vi "TDMS Read Telemtry Data.vi"() -> ()   [LabVIEW 2021]
doc: "This example demonstrates how to read measured data, text and timestamps from a .tdms file using the TDMS API."
panel:
  out "Measured Data":waveform(dbl)[](graph)
  in  "Event Data":i32(listbox)=-1
  # "Overview: Demonstrates the use of the TDMS Read function to read measured data, text and timestamps from an existing .tdms file.\nInstructions:\n1. Make sure you have already run TDMS Write Events Data.vi.\n2. Run this VI.\n3. Delete the .tdms file (located at [LabVIEW Data]\\Example Events Data.tdms) when you are done."
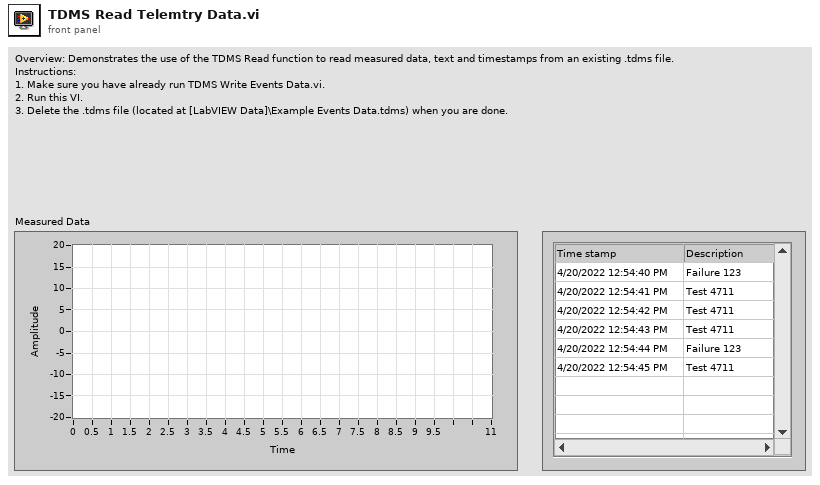
[diagram p1: front panel]
types:
  T1 = enum16{"open", "open or create", "create or replace", "create", "open (read-only)"}
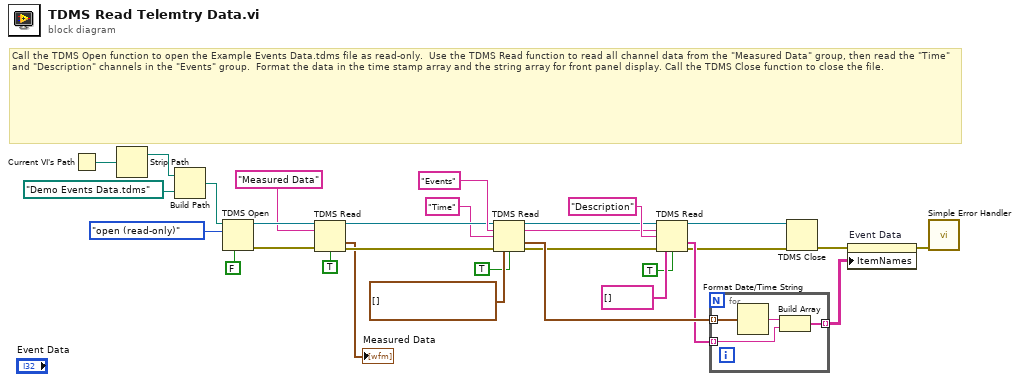
[diagram p0: block diagram]
diagram:
  # "Call the TDMS Open function to open the Example Events Data.tdms file as read-only.  Use the TDMS Read function to read all channel data from the \"Measured Data\" group, then read the \"Time\" and \"Description\" channels in the \"Events\" group.  Format the data in the time stamp array and the string array for front panel display. Call the TDMS Close function to close the file."
  n1 = Current VI's Path() -> (path=w2:path)
  n2 = Strip Path(path=w2) -> (stripped path=w1:path)  [unwired: 1 out]
  n3 = Build Path(base path=w1, name or relative path=path "Demo Events Data.tdms" ("file path")) -> (appended path=w14:path)
  n4 = TDMS Open(6:FALSE ("disable buffering (T)"), 10:T1."open (read-only)" ("operation"), 11:w14) -> (0:w27:errorcluster, 3:w28:refnum<k34>)  [unwired: 4 in]
  n5 = TDMS Read(0:w28, 5:"Measured Data" ("group name"), 11:w27, 13:TRUE ("return channels in file order? (F)")) -> (4:w24:refnum<k34>, 10:→"Measured Data":waveform(dbl)[], 15:w10:errorcluster)  [unwired: 4 in, 3 out]
  n6 = TDMS Read(0:w24, 5:"Events", 7:"Time", 11:w10, 12:timestamp[] [], 13:TRUE ("return channels in file order? (F)")) -> (4:w20:refnum<k34>, 6:w17:string, 10:w16:timestamp[], 15:w9:errorcluster)  [unwired: 2 in, 2 out]
  n7 = TDMS Read(0:w20, 5:w17, 7:"Description", 11:w9, 12:string[] [], 13:TRUE ("return channels in file order? (F)")) -> (4:w19:refnum<k34>, 10:w15:string[], 15:w8:errorcluster)  [unwired: 2 in, 3 out]
  n8 = for {
    tunnel: w16 -> [w34] mode=indexing
    tunnel: w15 -> [w32] mode=indexing
    tunnel: [w31] -> w6 mode=indexing
    n9 = Format Date/Time String(seconds (now)=w34) -> (date/time string=w33:string)  [unwired: 2 out]
    n10 = Build Array(w33, w32) -> (w31:string[])
  }
  n11 = TDMS Close(8:w8, 11:w19) -> (0:w5:errorcluster)  [unwired: 1 out]
  n12 = property on="Event Data" class="MCListbox (strict)"(error in=w5, "ItemNames"=w6) -> (error out=w4:errorcluster)  [unwired: 1 in, 1 out]
  n13 = call <vilib>:"Simple Error Handler.vi"("error in (no error)"=w4) -> ()  [unwired: 1 in, 8 out]
